vi "SubVI Tester.vi"() -> ()   [LabVIEW 2014]
panel:
  in  "최저 온도":dbl=10.0
  in  "최고 온도":dbl=30.0
  in  "정지":bool
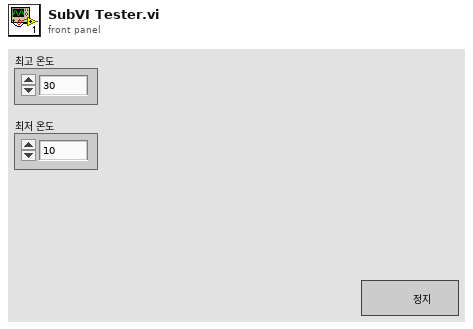
[diagram p1: front panel]
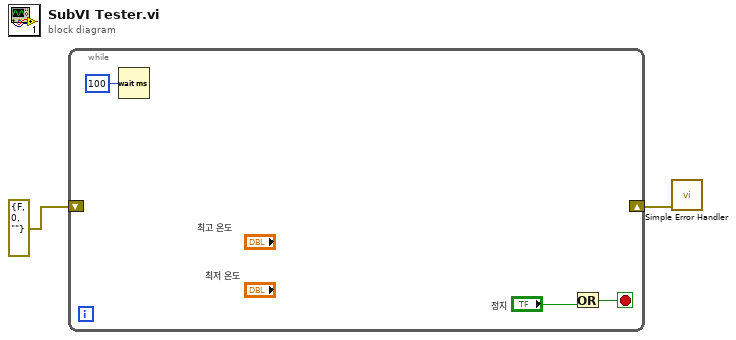
[diagram p0: block diagram]
diagram:
  n1 = while {
    shift-right: [_] -> w2
    shift-left: cluster{"상태":bool, "코드":i32, "소스":string} {"상태"=FALSE, "코드"=0, "소스"=""} ("에러 입력") -> [_]
    stop <- w3 stop-if-true
    n2 = Wait (ms)(milliseconds to wait=u32 100 ("대기 시간(ms)")) -> ()  [unwired: 1 out]
    n3 = Or(y="정지") -> (x .or. y?=w3:bool)  [unwired: 1 in]
  }
  n4 = call <vilib>:"Simple Error Handler.vi"("error in (no error)"=w2) -> ()  [unwired: 4 in, 5 out]
